vi "calculate max.vi"(10 "data input":dbl[](array[numeric])) -> (2 "top level":dbl format="%.3f")   [LabVIEW 2020]
uses:
  <vilib>/Analysis/baseanly.llb/Mean (DBL).vi
  <vilib>/Analysis/NI_AALBase.lvlib
panel:
  out "min value":dbl
  out "max value":dbl
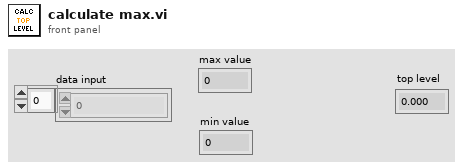
[diagram p1: front panel]
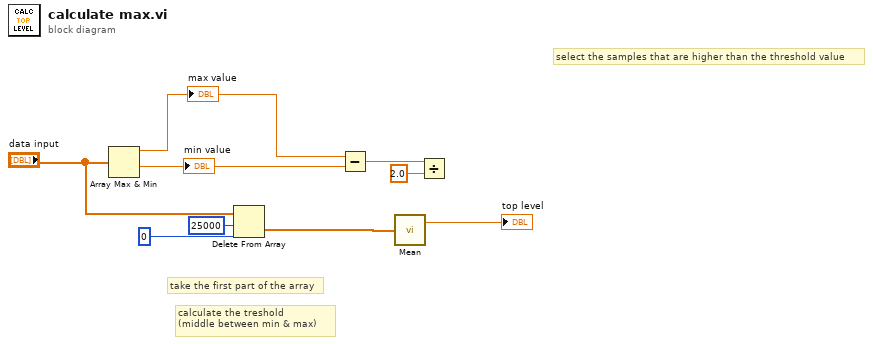
[diagram p0: block diagram]
diagram:
  # "calculate the treshold \n(middle between min & max)"
  # "select the samples that are higher than the threshold value"
  # "take the first part of the array"
  n1 = Array Max & Min(array="data input") -> (max value=w9:dbl, min value=w8:dbl)  [unwired: 2 out]
  "max value" <- w9
  "min value" <- w8
  n2 = Delete From Array(array="data input", length=25000, index=0) -> (deleted portion=w2:dbl[])  [unwired: 1 out]
  n3 = Subtract(x=w9, y=w8) -> (x-y=w7:dbl)
  n4 = call-poly <vilib>:"Mean.vi"("X"=w2) -> ("mean"=→"top level":dbl)  [unwired: 1 out]
  n5 = Divide(x=w7, y=2.0) -> ()  [unwired: 1 out]
